vi "Breadth First Search.vi"() -> ()   [LabVIEW 2014]
uses:
  ctl/Coin data--cluster.ctl
  ctl/Comparison result--enum.ctl
  OpenG/Reverse 2D Array (Boolean)__ogtk.vi
panel:
  out "Result":string
  out "Finished message":string
  out "Goal amount":dbl=7.0 format="£%#_g"
  out "No. solutions found":i32
  out "Total left in tree":dbl format="£%.2g"
  in  "Stop":bool
  out "Total of coins selected":dbl format="£%#.2g"
  out "Coins":bool[](array[boolean])
  out "Solutions found":bool[][](array[boolean])
  # "Beer Money"
  # "Breadth-First Search Solution"
  # "What's going on?\n\nThe algorithm is doing a breadth first search of the tree.\n\nIf the result is below the goal amount, it adds it to a list to come back to later. If the result is above the goal amount, it moves the lowest value coin to the next smallest denomination.\n\nIt is seriously slow - you won't get to the end unless you have a supercomputer. Make use of the stop button.\n\nTheoretically it can check every permutation and it finds the correct solution for smaller problems."
  # "1p"
  # "2p"
  # "5p"
  # "10p"
  # "20p"
  # "50p"
  # "£1"
  # "£2"
  # "£5"
  # "£10"
  # "Link to better explanation:\n\nhttps://youtu.be/z-Rf1_xs25s"
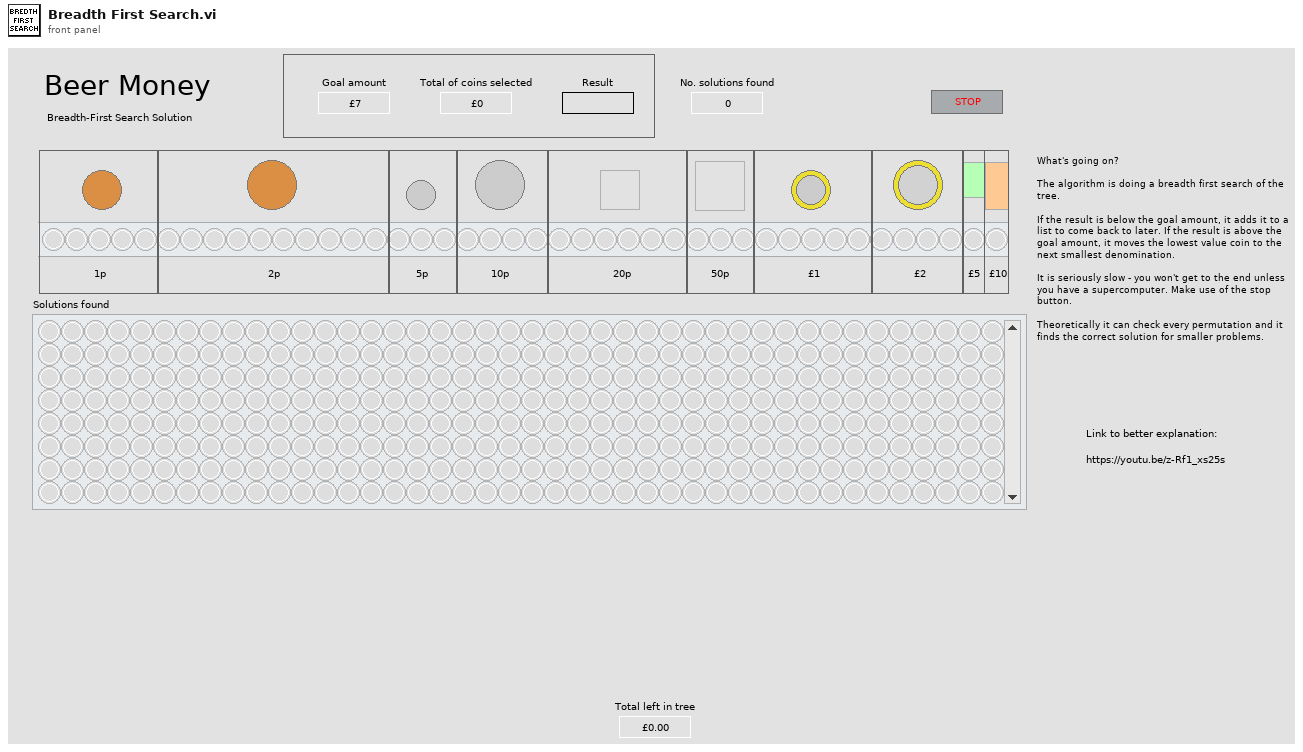
[diagram p1: front panel]
types:
  T1 = typedef "Coin data--cluster.ctl" = cluster{"Coin/note":i32, "Quantity":i32}
  T2 = cluster{"Wallet contents":T1[], "All my coins (values, £)":dbl[], "Indexes of next denom":i32[], "Wallet total (£)":dbl, "Index":i32, "Goal amount (£)":dbl, "No. coins":i32, "Coins State Cache":bool[], "Successful combos":bool[][], "'Hold' list (unexplored)":bool[][]}
  T3 = typedef "Comparison result--enum.ctl" = enum16{"Under", "Bingo!", "Over"}
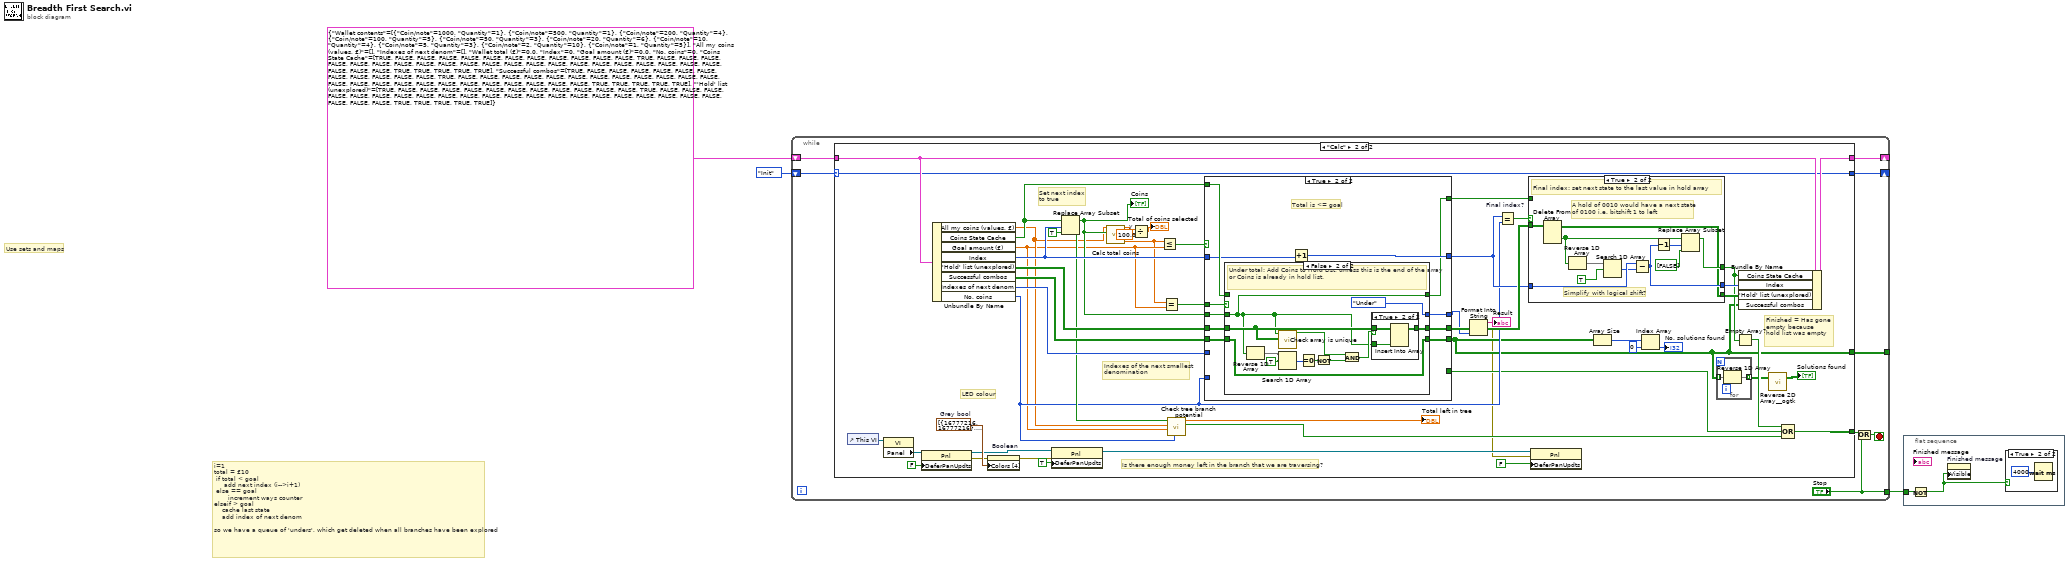
[diagram p0: block diagram]
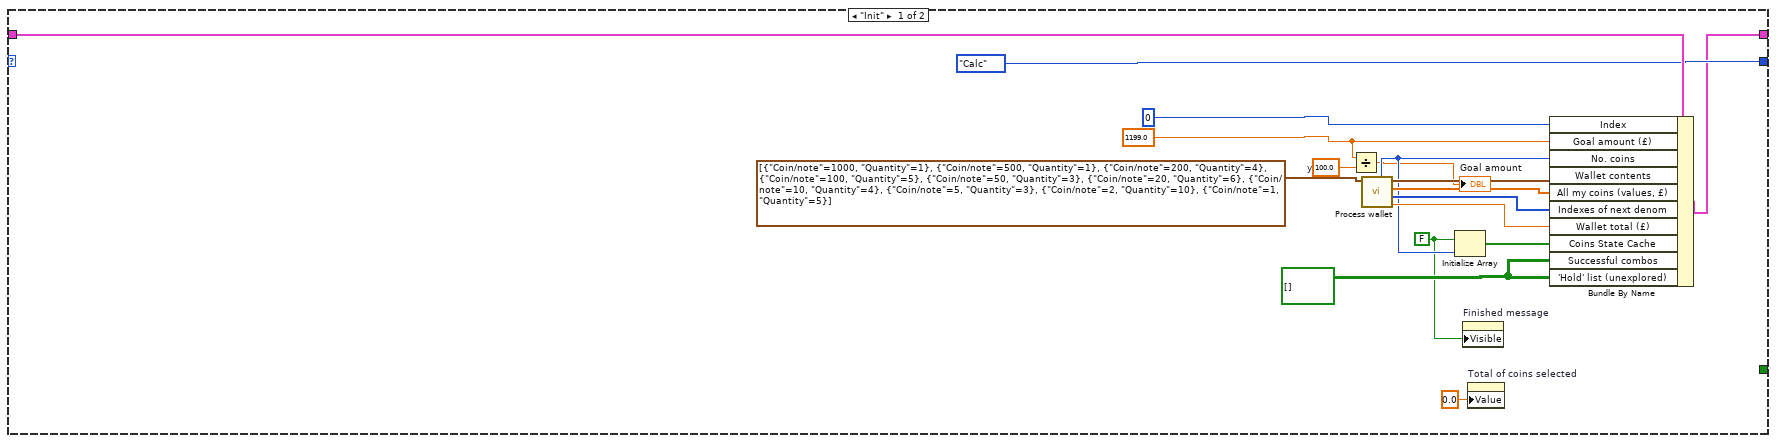
[diagram p3: hidden frame]
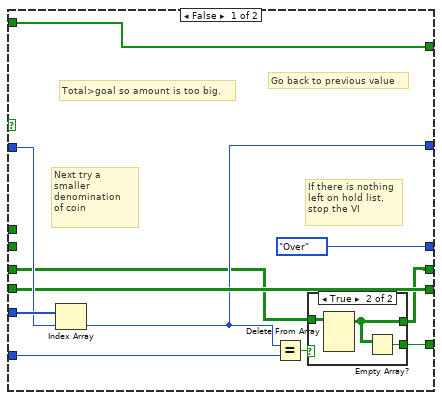
[diagram p5: hidden frame]
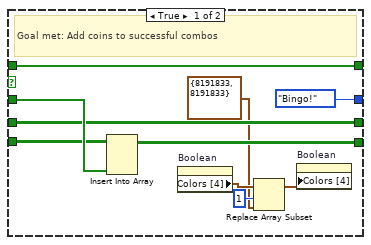
[diagram p7: hidden frame]
diagram:
  # "For a given index, what is the index of the next\nsmallest coin?"
  # "Total number of coins in wallet (const)"
  # "Array index of coin that we are examining"
  # "i=1\ntotal = £10\n if total < goal\n     add next index (i-->i+1)\n else == goal\n       increment ways counter\nelseif > goal\n    cache last state\n    add index of next denom\n\nso we have a queue of 'unders', which get deleted when all branches have been explored"
  # "Use sets and maps"
  n1 = while {
    shift-right: [w10] -> _
    shift-left: T2 {"Wallet contents"=[{"Coin/note"=1000, "Quantity"=1}, {"Coin/note"=500, "Quantity"=1}, {"Coin/note"=200, "Quantity"=4}, {"Coin/note"=100, "Quantity"=5}, {"Coin/note"=50, "Quantity"=3}, {"Coin/note"=20, "Quantity"=6}, {"Coin/note"=10, "Quantity"=4}, {"Coin/note"=5, "Quantity"=3}, {"Coin/note"=2, "Quantity"=10}, {"Coin/note"=1, "Quantity"=5}], "All my coins (values, £)"=[], "Indexes of next denom"=[], "Wallet total (£)"=0.0, "Index"=0, "Goal amount (£)"=0.0, "No. coins"=0, "Coins State Cache"=[TRUE, FALSE, FALSE, FALSE, FALSE, FALSE, FALSE, FALSE, FALSE, FALSE, FALSE, FALSE, TRUE, FALSE, FALSE, FALSE, FALSE, FALSE, FALSE, FALSE, FALSE, FALSE, FALSE, FALSE, FALSE, FALSE, FALSE, FALSE, FALSE, FALSE, FALSE, FALSE, FALSE, FALSE, FALSE, FALSE, FALSE, TRUE, TRUE, TRUE, TRUE, TRUE], "Successful combos"=[[TRUE, FALSE, FALSE, FALSE, FALSE, FALSE, FALSE, FALSE, FALSE, FALSE, FALSE, FALSE, TRUE, FALSE, FALSE, FALSE, FALSE, FALSE, FALSE, FALSE, FALSE, FALSE, FALSE, FALSE, FALSE, FALSE, FALSE, FALSE, FALSE, FALSE, FALSE, FALSE, FALSE, FALSE, FALSE, FALSE, FALSE, TRUE, TRUE, TRUE, TRUE, TRUE]], "'Hold' list (unexplored)"=[[TRUE, FALSE, FALSE, FALSE, FALSE, FALSE, FALSE, FALSE, FALSE, FALSE, FALSE, FALSE, TRUE, FALSE, FALSE, FALSE, FALSE, FALSE, FALSE, FALSE, FALSE, FALSE, FALSE, FALSE, FALSE, FALSE, FALSE, FALSE, FALSE, FALSE, FALSE, FALSE, FALSE, FALSE, FALSE, FALSE, FALSE, TRUE, TRUE, TRUE, TRUE, TRUE]]} -> [w11]
    shift-right: [w8] -> _
    shift-left: enum16{"Init", "Calc"}."Init" -> [w9]
    tunnel: [w6] -> _
    tunnel: ["Stop"] -> w1
    stop <- w5 stop-if-true
    n2 = case shown="\"Calc\"" w9 {
      selector: w9 -> [_ w70]
      tunnel: w11 -> [w28 w76]
      tunnel: [w19 w77] -> w10
      tunnel: [_ w54] -> w7
      tunnel: [enum16{"Init", "Calc"}."Calc" w70] -> w8
      tunnel: [_ w48] -> w6
      frame "Init" {
        w13 = 100.0  # y
        w17 = FALSE
        w14 = 1199.0 ("goal amount")
        w27 = bool[][] [] ("'Hold' list (unexplored)")
        n3 = Divide(x=w14, y=w13) -> (x/y=→"Goal amount":dbl)
        n4 = call "Process wallet.vi"("Wallet contents"=T1[] [{"Coin/note"=1000, "Quantity"=1}, {"Coin/note"=500, "Quantity"=1}, {"Coin/note"=200, "Quantity"=4}, {"Coin/note"=100, "Quantity"=5}, {"Coin/note"=50, "Quantity"=3}, {"Coin/note"=20, "Quantity"=6}, {"Coin/note"=10, "Quantity"=4}, {"Coin/note"=5, "Quantity"=3}, {"Coin/note"=2, "Quantity"=10}, {"Coin/note"=1, "Quantity"=5}]) -> ("Wallet total (£)"=w22:dbl, "Indexes of next denom"=w23:i32[], "All my coins (values, £)"=w24:dbl[], "Wallet contents (dup)"=w25:T1[], "No. coins"=w18:i32)  [unwired: 6 in]
        n5 = Initialize Array(w17, w18) -> (w21:bool[])
        n6 = property on="Finished message" class="Str"("Visible"=w17) -> ()  [unwired: 2 in, 2 out]
        n7 = property on="Total of coins selected" class="DigNum (strict)"("Value"=0.0 ("Total of coins selected")) -> ()  [unwired: 2 in, 2 out]
        n8 = Bundle By Name(cluster=w28, "Index"=0, "Goal amount (£)"=w14, "No. coins"=w18, "Wallet contents"=w25, "All my coins (values, £)"=w24, "Indexes of next denom"=w23, "Wallet total (£)"=w22, "Coins State Cache"=w21, "Successful combos"=w27, "'Hold' list (unexplored)"=w27) -> (w19:T2)
      }
      frame "Calc" {
        w30 = 100.0  # y
        w44 = cluster{u32, u32}[] [{16777216, 16777216}, {8026746, 8026746}, {16777216, 16777216}, {4095788, 4095788}]  # Grey bool
        # "LED colour"
        # "Indexes of the next smallest\ndenomination"
        # "Is there enough money left in the branch that we are traversing?"
        # "Set next index to true"
        # "Finished = Has gone empty because\nhold list was empty"
        n9 = control-ref of="This VI"() -> (w42:refnum<vi>)
        n10 = property class="VI"(reference=w42) -> ("Panel"=w41:refnum<vi>)  [unwired: 1 in, 2 out]
        n11 = property class="Pnl"(reference=w41, "DeferPanUpdts"=FALSE ("Defer Panel Updates")) -> (reference out=w38:refnum<vi>, error out=w35:errorcluster)  [unwired: 1 in]
        n12 = Unbundle By Name(w76) -> ("All my coins (values, £)"=w57:dbl[], "Coins State Cache"=w60:bool[], "Goal amount (£)"=w55:dbl, "Index"=w66:i32, "'Hold' list (unexplored)"=w73:bool[][], "Successful combos"=w72:bool[][], "Indexes of next denom"=w71:i32[], "No. coins"=w58:i32)
        n13 = property on="Boolean" class="Bool (strict)"(error in=w35, "Colors [4]"=w44) -> (error out=w37:errorcluster)  [unwired: 1 in, 1 out]
        n14 = property class="Pnl"(reference=w38, error in=w37, "DeferPanUpdts"=TRUE ("Defer Panel Updates")) -> (reference out=w34:refnum<vi>)  [unwired: 1 out]
        n15 = Replace Array Subset(array=w60, new element=TRUE ("new element/subarray"), index=w66) -> (w59:bool[])
        "Coins" <- w59
        n16 = call "Calc total coins.vi"("Coins"=w59, "All my coins"=w57) -> ("Total (£)"=w31:dbl)  [unwired: 9 in]
        n17 = Divide(x=w31, y=w30) -> (x/y=→"Total of coins selected":dbl)
        n18 = Less Or Equal?(x=w31, y=w55) -> (x <= y?=w75:bool)
        n19 = Equal?(x=w31, y=w55) -> (x = y?=w74:bool)
        n20 = call "Check tree branch potential.vi"("No. coins"=w58, "Goal amount"=w55, "All my coins"=w57, "Coins State Cache"=w59) -> ("Stop?"=w53:bool, "Total (£)"=→"Total left in tree":dbl)  [unwired: 6 in]
        n21 = case "Goal amount exceeded?" shown="True" w75 {
          tunnel: w74 -> [_ w109]
          tunnel: w66 -> [w103 w110]
          tunnel: [w99 w119] -> w63
          tunnel: w59 -> [_ w115]
          tunnel: w73 -> [w98 w118]
          tunnel: w72 -> [w102 w117]
          tunnel: [w102 w116] -> w48
          tunnel: [w97 w114] -> w67
          tunnel: w71 -> [w104 _]
          tunnel: [w95 w112] -> w68
          tunnel: w58 -> [w100 _]
          tunnel: [w96 _] -> w52
          tunnel: w60 -> [w95 w111]
          tunnel: [Comparison_result--enum."Over" ("Total") w113] -> w40
          frame False {
            # "If there is nothing\nleft on hold list,\nstop the VI"
            # "Go back to previous value"
            # "Next try a smaller denomination\nof coin"
            # "Total>goal so amount is too big."
            n22 = Index Array(array=w104, index=w103) -> (element=w99:i32)
            n23 = Equal?(x=w99, y=w100) -> (x = y?=w101:bool)
            n24 = case shown="True" w101 {
              tunnel: [w105 w107] -> w97
              tunnel: w98 -> [w105 w108]
              tunnel: [_ w106] -> w96
              frame False {
              }
              frame True {
                n25 = Delete From Array(array=w108) -> (array with subset deleted=w107:bool[][])  [unwired: 3 in, 1 out]
                n26 = Empty Array?(array=w107) -> (empty?=w106:bool)
              }
            }
          }
          frame True {
            # "Total is <= goal"
            n27 = case shown="False" w109 {
              tunnel: w118 -> [w126 w138]
              tunnel: w117 -> [w128 w140]
              tunnel: [w127 w140] -> w116
              tunnel: w115 -> [w129 w130]
              tunnel: [w126 w141] -> w114
              tunnel: [Comparison_result--enum."Bingo!" ("Total") Comparison_result--enum."Under" ("Total")] -> w113
              tunnel: [w124 w130] -> w112
              tunnel: w111 -> [w124 _]
              frame True {
                # "Goal met: Add coins to successful combos"
                n28 = Insert Into Array(array=w128, new element=w129) -> (w127:bool[][])  [unwired: 2 in]
                n29 = property on="Boolean" class="Bool (strict)"() -> ("Colors [4]"=w123:cluster{u32, u32}[])  [unwired: 2 in, 2 out]
                n30 = Replace Array Subset(array=w123, new element=cluster{u32, u32} {8191833, 8191833} ("new element/subarray"), index=1) -> (w121:cluster{u32, u32}[])
                n31 = property on="Boolean" class="Bool (strict)"("Colors [4]"=w121) -> ()  [unwired: 2 in, 2 out]
              }
              frame False {
                # "Under total: Add Coins to Hold List, unless this is the end of the array or Coins is already in hold list."
                n32 = Reverse 1D Array(array=w130) -> (reversed array=w134:bool[])
                n33 = call "Check array is unique.vi"("'Hold' list"=w138, "Coins State Cache"=w130) -> ("Is unique?"=w137:bool)  [unwired: 9 in]
                n34 = Search 1D Array(1D array=w134, element=TRUE) -> (index of element=w133:i32)  [unwired: 1 in]
                n35 = Equal To 0?(x=w133) -> (x = 0?=w132:bool)
                n36 = Not(x=w132) -> (.not. x?=w131:bool)
                n37 = And(x=w137, y=w131) -> (x .and. y?=w136:bool)
                n38 = case shown="True" w136 {
                  tunnel: [w142 w145] -> w141
                  tunnel: w138 -> [w142 w144]
                  tunnel: w130 -> [_ w143]
                  frame False {
                  }
                  frame True {
                    n39 = Insert Into Array(array=w144, new element=w143) -> (w145:bool[][])  [unwired: 2 in]
                  }
                }
              }
            }
            n40 = Increment(x=w110) -> (x+1=w119:i32)
          }
        }
        n41 = Format Into String(w40) -> (resulting string=→"Result":string, error out=w32:errorcluster)  [unwired: 3 in]
        n42 = Equal? "Final index?"(x=w63, y=w58) -> (x = y?=w69:bool)
        n43 = case shown="True" w69 {
          tunnel: w67 -> [w81 w89]
          tunnel: [w82 w91] -> w61
          tunnel: w68 -> [w82 _]
          tunnel: [w81 w90] -> w62
          tunnel: [w80 w92] -> w64
          tunnel: w63 -> [w80 w93]
          frame False {
            # "Not final index - do nothing"
          }
          frame True {
            # "Simplify with logical shift?"
            # "A hold of 0010 would have a next state\nof 0100 i.e. bitshift 1 to left"
            # "Final index: set next state to the last value in hold array"
            n44 = Delete From Array(array=w89) -> (deleted portion=w85:bool[], array with subset deleted=w90:bool[][])  [unwired: 3 in]
            n45 = Reverse 1D Array(array=w85) -> (reversed array=w86:bool[])
            n46 = Search 1D Array(1D array=w86, element=TRUE) -> (index of element=w83:i32)  [unwired: 1 in]
            n47 = Subtract(x=w93, y=w83) -> (x-y=w92:i32)
            n48 = Decrement(x=w92) -> (x-1=w84:i32)
            n49 = Replace Array Subset(array=w85, new element=bool[] [FALSE] ("new element/subarray"), index=w84) -> (w91:bool[])
          }
        }
        n50 = property class="Pnl"(reference=w34, error in=w32, "DeferPanUpdts"=FALSE ("Defer Panel Updates")) -> ()  [unwired: 2 out]
        n51 = Array Size(array=w48) -> (size(s)=w50:i32[])
        n52 = Index Array(array=w50, index=0) -> (element=→"No. solutions found":i32)
        n53 = for {
          tunnel: w48 -> [w79] mode=indexing
          tunnel: [w78] -> w46 mode=indexing
          n54 = Reverse 1D Array(array=w79) -> (reversed array=w78:bool[])
        }
        n55 = Empty Array?(array=w61) -> (empty?=w51:bool)
        n56 = Bundle By Name(cluster=w76, "Coins State Cache"=w61, "Index"=w64, "'Hold' list (unexplored)"=w62, "Successful combos"=w48) -> (w77:T2)
        n57 = call-poly "Reverse 2D Array__ogtk.vi"("Array"=w46) -> ("Reversed Array"=→"Solutions found":bool[][])  [unwired: 2 in]
        n58 = Compound Arithmetic op=OR(w51, w52, w53) -> (w54:bool)
      }
    }
    n59 = Or(x=w7, y="Stop") -> (x .or. y?=w5:bool)
  }
  n60 = flat-sequence {
    tunnel: w1 -> [w147]
    frame #0 {
      n61 = Not(x=w147) -> (.not. x?=w146:bool)
      n62 = property on="Finished message" class="Str"("Visible"=w146) -> ()  [unwired: 2 in, 2 out]
      n63 = case shown="True" w146 {
        frame False {
        }
        frame True {
          n64 = Wait (ms)(milliseconds to wait=u32 4000) -> ()  [unwired: 1 out]
        }
      }
    }
  }
